vi "Begin.vi"() -> (0 "error out":errorcluster)   [LabVIEW 2019]
doc: "Called before other user functions, this VI is expected to open initial I/O refnums, load in file data, and do all program initialization. Notice that the <B>error out</B> terminal is simply used for data flow. Wiring it to other structures or subVIs ensures that this VI runs first."
uses:
  <vilib>/Rock Robotics/WPI/DriverStation/WPI_DriverStationRobotMode2.ctl
  <vilib>/Rock Robotics/WPI/ThirdParty/Phoenix-LabVIEW/Motor Controller/Controls/CTRE_Phoenix_MotorControl_SupplyCurrentLimitConfiguration.ctl
  Robot Global Data.vi
panel:
  in  "Accelerator Follower CAN ID":u8=23
  in  "Flywheel Follwer CAN ID":u8=46
  in  "Accelerator Enable Follower":bool
  in  "Flywheel Enable Follower":bool
  in  "Flywheel Leader CAN ID":u8=7
  in  "Accelerator Leader CAN ID":u8=23
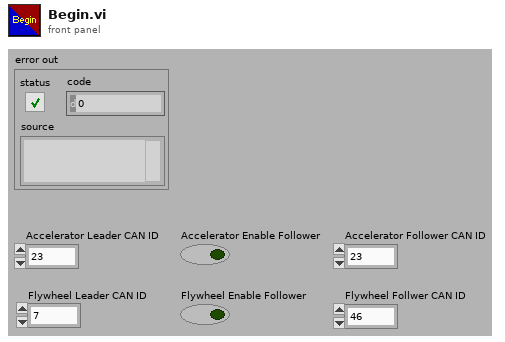
[diagram p1: front panel]
types:
  T1 = typedef "CTRE_Phoenix_MotorControl_SupplyCurrentLimitConfiguration.ctl" = cluster{"Enable?":bool, "Current Limit":dbl, "Threshold Current":dbl, "Threshold Time":dbl}
  T2 = typedef "WPI_DriverStationRobotMode2.ctl" = enum16{"Autonomous Disabled", "Autonomous Enabled", "Teleop Disabled", "Teleop Enabled", "Disconnected", "Finish", "Test Disabled", "Test Enabled", "Emergency Stopped"}
  T3 = typedef "WPI_MotorControlDeviceRef.ctl" = cluster{"DeviceStatus":errorcluster, "Type":T4, "PWM":cluster{"PWM Channel":T5, "DeadBand":T6}, "CAN":cluster{"Device Number":u8, "SetOutput VI Ref":variant, "GetOutput VI Ref":variant, "Enable VI Ref":variant, "Disable VI Ref":variant, "Data":variant}, "Invert":bool, "DIO PWM":cluster{"PWM \"Enable\" Channel":T5, "DIOChannel":T7, "PWM Rate":dbl}}
  T4 = typedef "WPI_MotorControlType.ctl" = enum16{"PWM", "CAN", "DIO PWM"}
  T5 = typedef "FPGA_DIOPWMChannel.ctl" = enum8{"PWM 0", "PWM 1", "PWM 2", "PWM 3", "PWM 4", "PWM 5", "PWM 6", "PWM 7", "PWM 8", "PWM 9", "PWM MXP 0", "PWM MXP 1", "PWM MXP 2", "PWM MXP 3", "PWM MXP 4", "PWM MXP 5", "PWM MXP 6", "PWM MXP 7", "PWM MXP 8", "PWM MXP 9", "Invalid"}
  T6 = typedef "WPI_PWMDeadband.ctl" = cluster{"Name":string, "maxPositivePwm":i32, "minPositivePwm":i32, "centerPwm":i32, "maxNegativePwm":i32, "minNegativePwm":i32, "angularRange":u16}
  T7 = typedef "FPGA_DIOChannel.ctl" = enum8{"DIO 0", "DIO 1", "DIO 2", "DIO 3", "DIO 4", "DIO 5", "DIO 6", "DIO 7", "DIO 8", "DIO 9", "DIO MXP 0", "DIO MXP 1", "DIO MXP 2", "DIO MXP 3", "DIO MXP 4", "DIO MXP 5", "DIO MXP 6", "DIO MXP 7", "DIO MXP 8", "DIO MXP 9", "DIO MXP 10", "DIO MXP 11", "DIO MXP 12", "DIO MXP 13", "DIO MXP 14", "DIO MXP 15", "SPI Port CS1", "SPI Port CS2", "SPI Port CS3", "SPI Port MISO", "SPI Port MOSI", "Invalid"}
  T8 = enum16{"FollowerType_PercentOutput", "FollowerType_AuxOutput1"}
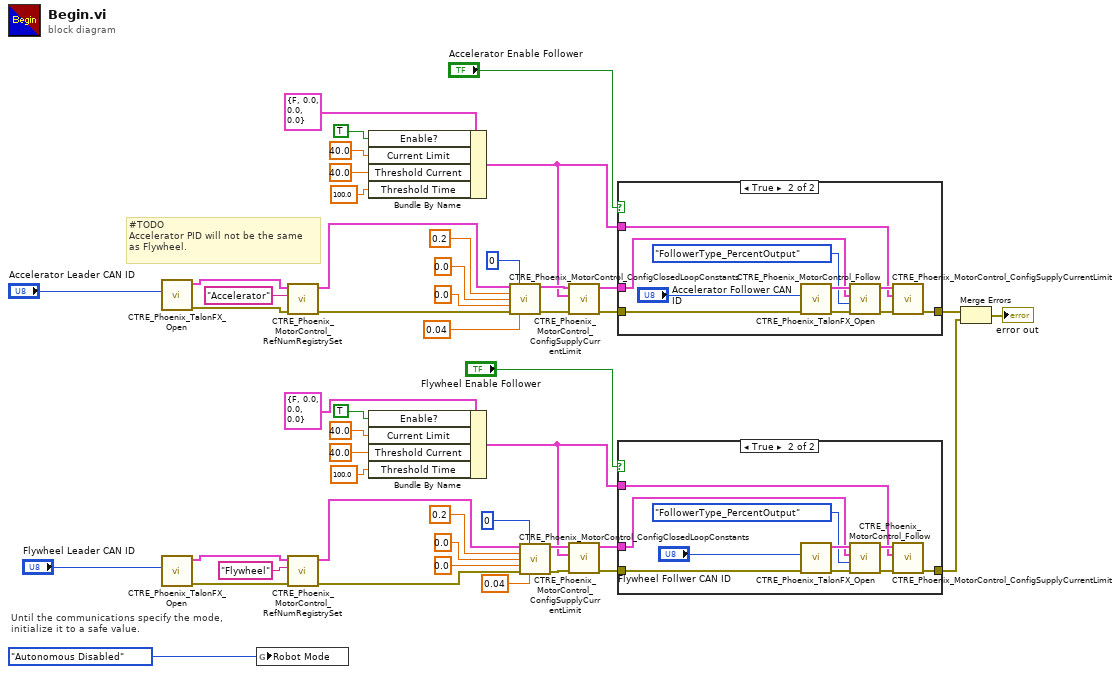
[diagram p0: block diagram]
diagram:
  # "#TODO\nAccelerator PID will not be the same\nas Flywheel."
  # "Until the communications specify the mode,\ninitialize it to a safe value."
  n1 = call <vilib>:"CTRE_Phoenix_TalonFX_Open.vi"("Device Number"="Accelerator Leader CAN ID") -> ("error out"=w30:errorcluster, "CAN Talon SRX Ref"=w46:T3)  [unwired: 9 in]
  n2 = call <vilib>:"CTRE_Phoenix_TalonFX_Open.vi"("Device Number"="Flywheel Leader CAN ID") -> ("error out"=w31:errorcluster, "CAN Talon SRX Ref"=w44:T3)  [unwired: 9 in]
  n3 = global write "Robot Global Data.vi" "Robot Mode"(WPI_DriverStationRobotMode2."Autonomous Disabled" ("Robot Mode")) -> ()
  n4 = call <vilib>:"CTRE_Phoenix_MotorControl_RefNumRegistrySet.vi"("error in (no error)"=w30, "refnum name"="Accelerator", "PhoenixMotorControlDevRef"=w46) -> ("error out"=w29:errorcluster, "PhoenixMotorControlDevRef"=w34:T3)  [unwired: 7 in]
  n5 = call <vilib>:"CTRE_Phoenix_MotorControl_RefNumRegistrySet.vi"("error in (no error)"=w31, "refnum name"="Flywheel", "PhoenixMotorControlDevRef"=w44) -> ("error out"=w32:errorcluster, "PhoenixMotorControlDevRef"=w33:T3)  [unwired: 7 in]
  n6 = Bundle By Name(cluster=T1 {"Enable?"=FALSE, "Current Limit"=0.0, "Threshold Current"=0.0, "Threshold Time"=0.0} ("Supply Current Limit Configuration"), "Enable?"=TRUE, "Current Limit"=40.0, "Threshold Current"=40.0, "Threshold Time"=100.0) -> (w1:T1)
  n7 = Bundle By Name(cluster=T1 {"Enable?"=FALSE, "Current Limit"=0.0, "Threshold Current"=0.0, "Threshold Time"=0.0} ("Supply Current Limit Configuration"), "Enable?"=TRUE, "Current Limit"=40.0, "Threshold Current"=40.0, "Threshold Time"=100.0) -> (w14:T1)
  n8 = call <vilib>:"CTRE_Phoenix_MotorControl_ConfigClosedLoopConstants.vi"("PhoenixMotorControlDevRef"=w34, "slotIdx"=0, "P"=0.2, "I"=0.0, "D"=0.0, "error in (no error)"=w29, "F"=0.04) -> ("PhoenixMotorControlDevRef"=w11:T3, "error out"=w10:errorcluster)  [unwired: 7 in]
  n9 = call <vilib>:"CTRE_Phoenix_MotorControl_ConfigClosedLoopConstants.vi"("PhoenixMotorControlDevRef"=w33, "slotIdx"=0, "P"=0.2, "I"=0.0, "D"=0.0, "error in (no error)"=w32, "F"=0.04 ("I")) -> ("PhoenixMotorControlDevRef"=w18:T3, "error out"=w17:errorcluster)  [unwired: 7 in]
  n10 = call <vilib>:"CTRE_Phoenix_MotorControl_ConfigSupplyCurrentLimit.vi"("error in (no error)"=w10, "Supply Current Limit Configuration"=w1, "PhoenixMotorControlDevRef"=w11) -> ("error out"=w8:errorcluster, "PhoenixMotorControlDevRef"=w7:T3)  [unwired: 7 in]
  n11 = call <vilib>:"CTRE_Phoenix_MotorControl_ConfigSupplyCurrentLimit.vi"("error in (no error)"=w17, "Supply Current Limit Configuration"=w14, "PhoenixMotorControlDevRef"=w18) -> ("error out"=w15:errorcluster, "PhoenixMotorControlDevRef"=w16:T3)  [unwired: 7 in]
  n12 = case shown="True" "Accelerator Enable Follower" {
    tunnel: w7 -> [_ w57]
    tunnel: w8 -> [w49 w54]
    tunnel: [w49 w51] -> w9
    tunnel: w1 -> [_ w50]
    frame False {
    }
    frame True {
      n13 = call <vilib>:"CTRE_Phoenix_TalonFX_Open.vi"("error in"=w54, "Device Number"="Accelerator Follower CAN ID") -> ("error out"=w55:errorcluster, "CAN Talon SRX Ref"=w58:T3)  [unwired: 8 in]
      n14 = call <vilib>:"CTRE_Phoenix_MotorControl_Follow.vi"("error in (no error)"=w55, "FollowerType"=T8."FollowerType_PercentOutput", "Master Controller to Follow"=w57, "PhoenixMotorControlDevRef"=w58) -> ("error out"=w52:errorcluster, "PhoenixMotorControlDevRef"=w53:T3)  [unwired: 6 in]
      n15 = call <vilib>:"CTRE_Phoenix_MotorControl_ConfigSupplyCurrentLimit.vi"("error in (no error)"=w52, "Supply Current Limit Configuration"=w50, "PhoenixMotorControlDevRef"=w53) -> ("error out"=w51:errorcluster)  [unwired: 7 in, 1 out]
    }
  }
  n16 = case shown="True" "Flywheel Enable Follower" {
    tunnel: w16 -> [_ w69]
    tunnel: w15 -> [w60 w65]
    tunnel: w14 -> [_ w62]
    tunnel: [w60 w61] -> w13
    frame False {
    }
    frame True {
      n17 = call <vilib>:"CTRE_Phoenix_TalonFX_Open.vi"("error in"=w65, "Device Number"="Flywheel Follwer CAN ID") -> ("error out"=w66:errorcluster, "CAN Talon SRX Ref"=w70:T3)  [unwired: 8 in]
      n18 = call <vilib>:"CTRE_Phoenix_MotorControl_Follow.vi"("error in (no error)"=w66, "FollowerType"=T8."FollowerType_PercentOutput", "Master Controller to Follow"=w69, "PhoenixMotorControlDevRef"=w70) -> ("error out"=w63:errorcluster, "PhoenixMotorControlDevRef"=w64:T3)  [unwired: 6 in]
      n19 = call <vilib>:"CTRE_Phoenix_MotorControl_ConfigSupplyCurrentLimit.vi"("error in (no error)"=w63, "Supply Current Limit Configuration"=w62, "PhoenixMotorControlDevRef"=w64) -> ("error out"=w61:errorcluster)  [unwired: 7 in, 1 out]
    }
  }
  n20 = Merge Errors(w9, w13) -> (→"error out":errorcluster)
